vi "UE9 Thermocouple Example.vi"(8 "error in":errorcluster) -> (0 "error out":errorcluster)   [LabVIEW 2021]
panel:
  in  "UE9-Pro":bool
  in  "Gain":dbl=1.0 format="%.4f"
  in  "Cold Junction Sensor Offset [degK]":dbl format="%.4f"
  in  "Cold Junction Sensor Slope [degK/V]":dbl=1.0 format="%.4f"
  in  "Cold Junction Sensor Channel":i32=133
  out "Temperatures (Deg C)":dbl[](array[numeric]) format="%.1f"
  out "Cold Junction\nTemperature (Deg C)":dbl format="%.2f"
  in  "Offset Voltages":dbl[](array[numeric])=[0.0, 0.0] format="%.6f"
  in  "Channels":i32[](array[numeric])=[0, 1]
  out "Raw Readings":dbl[](array[numeric]) format="%.6f"
  out "Error Message":string
  # "Uses the first found UE9 over USB.  Requires UD driver V2.60+.\n\nAquires multiple analog input channels and performs a K type thermocouple conversion on them.  For\nimproved accuracy, set the TCs near the UE9 so they are at the same ambient temperature and thus\nthe measured voltage should be zero.  With the UE9 powered-up, allow 20-60 minutes for everything\nto stabilize.  Then note the voltage offset in the \"Readings\" array, and enter this in the \"Offset\" array."
  # "If using an LJTIA (or other amplifier) to amplify the\nthermocouple voltages, enter the gain here."
  # "The voltage from a thermocouple corresponds to the temperature\ndifference between one end and the other.  To determine the temp\nat the remote end, we must know the temperature at the local end.\nThe local end is called the cold junction, and in this case is\nthe UE9/LJTIA.  Enter the channel # from which to read the cold\njuntion temperature, and enter the slope/offset required to convert\nthat temperature to degrees K."
  # "Internal Sensor = 133"
  # "Internal=1, EI-1022=100, EI-1034=55.56"
  # "Internal=0, EI-1022=0, EI-1034=255.37"
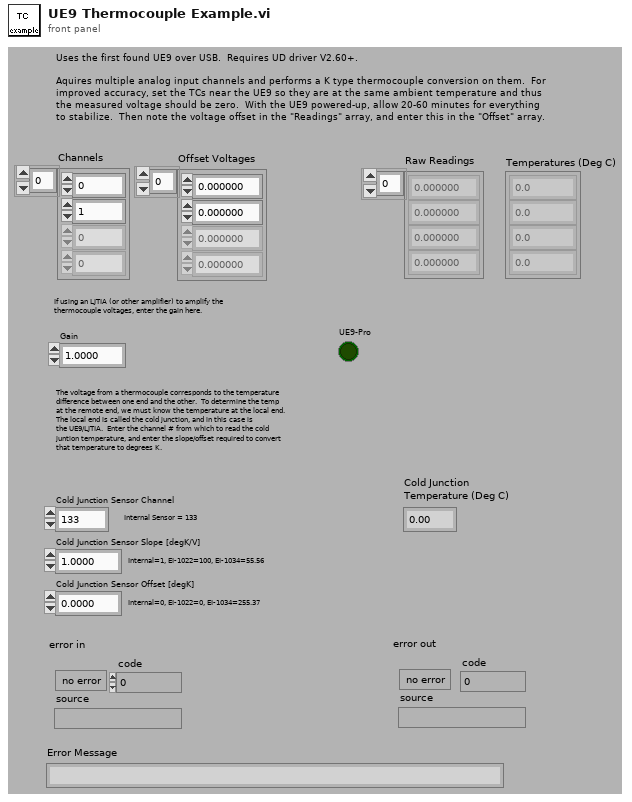
[diagram p1: front panel]
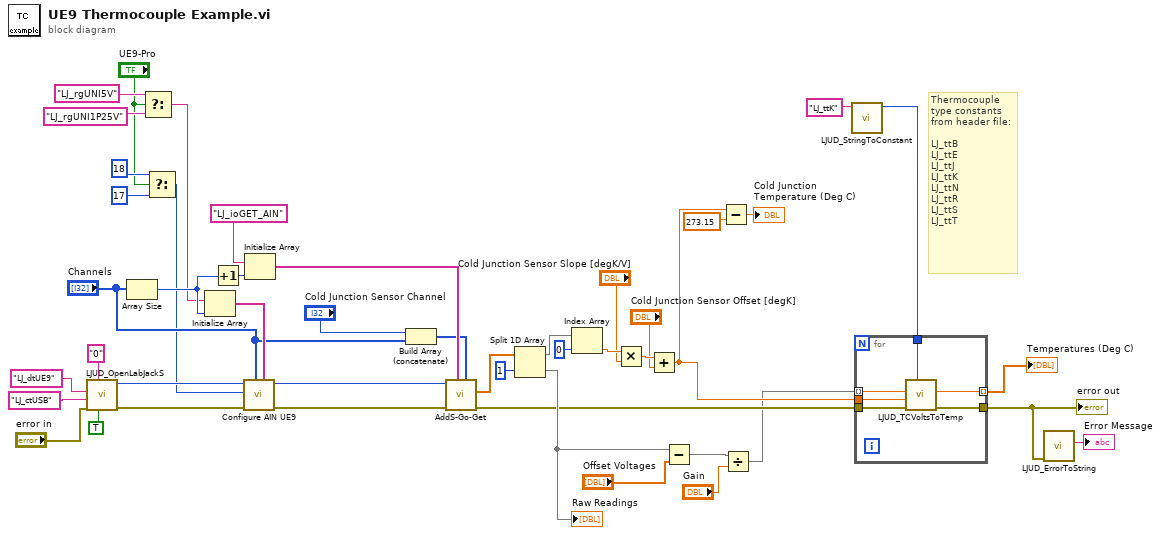
[diagram p0: block diagram]
diagram:
  # "Thermocouple\ntype constants\nfrom header file:\n\nLJ_ttB\nLJ_ttE\nLJ_ttJ\nLJ_ttK\nLJ_ttN\nLJ_ttR\nLJ_ttS\nLJ_ttT"
  n1 = call "LJUD_OpenLabJackS.vi"("FirstFound"=TRUE, "Address"="0", "error in"="error in", "ConnectionType"="LJ_ctUSB", "DeviceType"="LJ_dtUE9") -> ("error out"=w42:errorcluster, "Handle"=w39:i32)  [unwired: 4 in, 1 out]
  n2 = Array Size(array="Channels") -> (size(s)=w34:i32)
  n3 = Select(t="LJ_rgUNI5V" ("AIN Range"), s="UE9-Pro", f="LJ_rgUNI1P25V" ("AIN Range")) -> (s? t:f=w1:string)
  n4 = Select(t=18 ("Resolution"), s="UE9-Pro", f=17 ("Resolution")) -> (s? t:f=w2:i32)
  n5 = Initialize Array(w1, w34) -> (w36:string[])
  n6 = Increment(x=w34) -> (x+1=w35:i32)
  n7 = call "Configure AIN UE9.vi"("Ranges"=w36, "Channels"="Channels", "error in"=w42, "Resolution"=w2, "Handle In"=w39) -> ("error out"=w41:errorcluster, "Handle Out"=w40:i32)  [unwired: 5 in]
  n8 = Initialize Array("LJ_ioGET_AIN" ("IOType"), w35) -> (w37:string[])
  n9 = Build Array (concatenate)("Cold Junction Sensor Channel", "Channels") -> (w33:i32[])
  n10 = call "AddS-Go-Get.vi"("Channels"=w33, "IOTypes"=w37, "error in"=w41, "Handle In"=w40) -> ("error out"=w13:errorcluster, "Values Read"=w26:dbl[])  [unwired: 5 in, 1 out]
  n11 = Split 1D Array(array=w26, index=1) -> (first subarray=w25:dbl[], second subarray=w14:dbl[])
  "Raw Readings" <- w14
  n12 = Index Array(array=w25, index=0 ("Index")) -> (element=w23:dbl)
  n13 = Multiply(x=w23, y="Cold Junction Sensor Slope [degK/V]") -> (x*y=w22:dbl)
  n14 = Add(x=w22, y="Cold Junction Sensor Offset [degK]") -> (x+y=w12:dbl)
  n15 = Subtract(x=w14, y="Offset Voltages") -> (x-y=w15:dbl[])
  n16 = Subtract(x=w12, y=273.15) -> (x-y=→"Cold Junction\nTemperature (Deg C)":dbl)
  n17 = Divide(x=w15, y="Gain") -> (x/y=w11:dbl[])
  n18 = call "LJUD_StringToConstant.vi"("String"="LJ_ttK") -> ("Constant Number"=w10:i32)  [unwired: 9 in, 1 out]
  n19 = for {
    tunnel: w13 -> [w52]
    tunnel: w12 -> [w51]
    tunnel: w11 -> [w50] mode=indexing
    tunnel: w10 -> [w49]
    tunnel: [w48] -> w9
    tunnel: [w47] -> w8 mode=indexing
    n20 = call "LJUD_TCVoltsToTemp.vi"("TCType"=w49, "error in"=w52, "CJTempK"=w51, "TCVolts"=w50) -> ("error out"=w48:errorcluster, "TCTempC"=w47:dbl)  [unwired: 4 in, 2 out]
  }
  "error out" <- w9
  "Temperatures (Deg C)" <- w8
  n21 = call "LJUD_ErrorToString.vi"("error in"=w9) -> ("String"=→"Error Message":string)  [unwired: 10 in]
